vi "GetArray.vi"(8 "error in (no error)":errorcluster, 10 "size":i32, 11 "MsgPackDeserializer in":refnum<class "MsgPackDeserializer.lvclass">) -> (0 "error out":errorcluster, 2 "Variant":variant, 3 "MsgPackDeserializer out":refnum<class "MsgPackDeserializer.lvclass">)   [LabVIEW 2015, in "MsgPackDeserializer.lvclass"]
uses:
  MsgPackDeserializer.lvclass
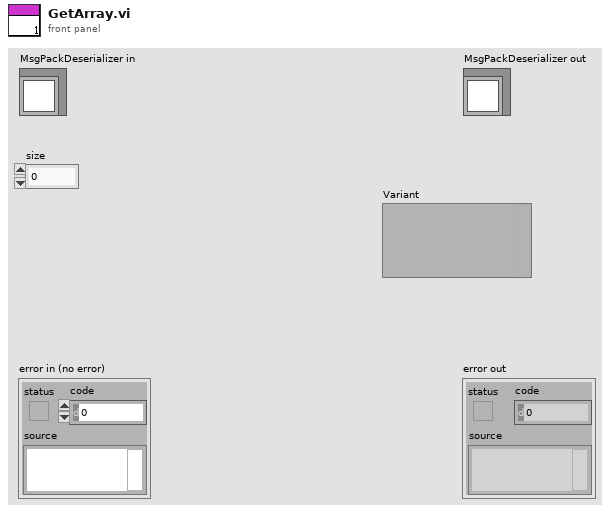
[diagram p1: front panel]
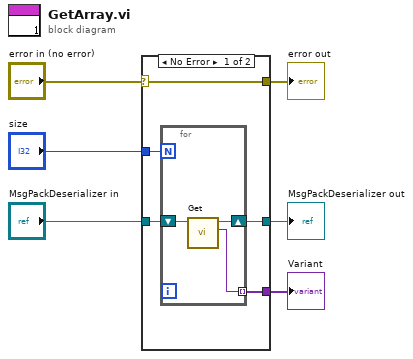
[diagram p0: block diagram]
diagram:
  n1 = case shown="No Error" "error in (no error)" {
    selector: "error in (no error)" -> [w11 w16]
    tunnel: [w11 w16] -> w5
    tunnel: [w9 w15] -> w3
    tunnel: "MsgPackDeserializer in" -> [w10 w15]
    tunnel: [w8 _] -> w2
    tunnel: "size" -> [w7 _]
    frame No Error {
      n2 = for {
        N: w7 -> [_]
        shift-right: [w13] -> w9
        shift-left: w10 -> [w14]
        tunnel: [w12] -> w8 mode=indexing
        n3 = call "Get.vi"("MsgPackDeserializer in"=w14) -> ("Variant"=w12:variant, "MsgPackDeserializer out"=w13:refnum<class "MsgPackDeserializer.lvclass">)  [unwired: 8 in, 1 out]
      }
    }
    frame Error {
    }
  }
  "error out" <- w5
  "MsgPackDeserializer out" <- w3
  "Variant" <- w2
